vi "4p1_HW_Task1_pipoat.vi"() -> ()   [LabVIEW 2016]
uses:
  <vilib>/express/express arith-compare/Formula/XNode/ExpressFormulaBlockNode.xnode
panel:
  in  "Height":dbl
  out "Height of Fish":dbl
  in  "glass thickness (ft)":dbl
  in  "human distance from glass (ft)":dbl
  in  "fish distance from glass (ft)":dbl
  in  "reflective index of water":dbl
  in  "reflective index of glass":dbl
  in  "reflective index of air":dbl
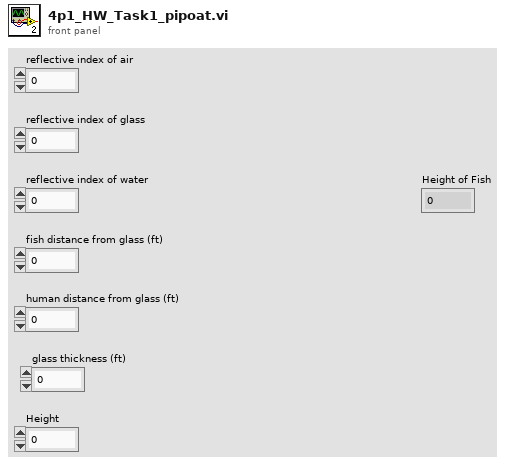
[diagram p1: front panel]
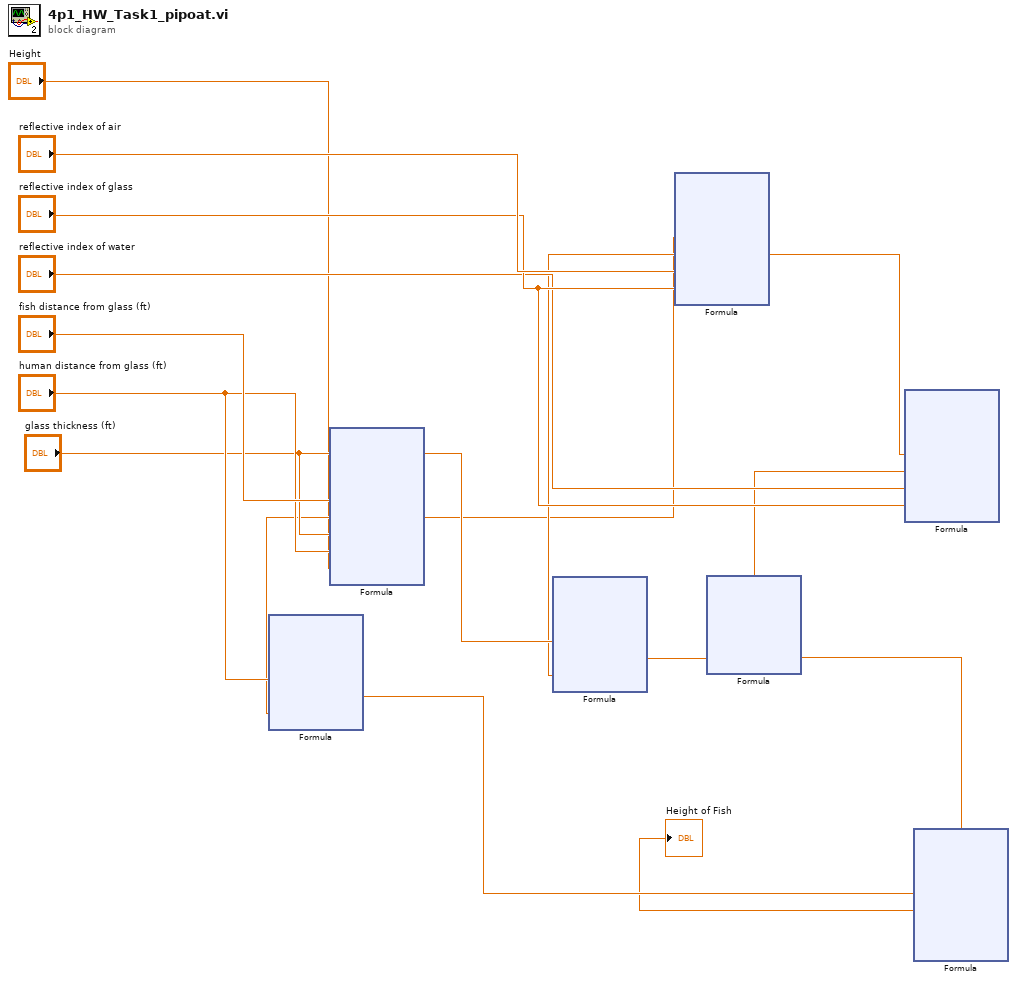
[diagram p0: block diagram]
diagram:
  n1 = xnode "Formula"("fish distance"="fish distance from glass (ft)", "glass thickness"="glass thickness (ft)", "human distance"="human distance from glass (ft)", "height"="Height") -> ("Result"=w2:dbl)  [unwired: 1 in, 1 out]
  n2 = xnode "Formula"("human distance"="human distance from glass (ft)", "tangent angle"=w2) -> ("Result"=w8:dbl)  [unwired: 1 in, 1 out]
  n3 = xnode "Formula"("tangent angle"=w2, "ref. index of air"="reflective index of air", "ref. index of glass"="reflective index of glass") -> ("Result"=w4:dbl)  [unwired: 1 in, 1 out]
  n4 = xnode "Formula"("glass thickness"="glass thickness (ft)", "angle B"=w4) -> ("Result"=w5:dbl)  [unwired: 1 in, 1 out]
  n5 = xnode "Formula"("Angle B"=w4, "ref. index of water"="reflective index of water", "ref. index of glass"="reflective index of glass") -> ("Result"=w3:dbl)  [unwired: 1 in, 1 out]
  n6 = xnode "Formula"("angle C"=w3) -> ("Result"=w7:dbl)  [unwired: 1 in, 1 out]
  n7 = xnode "Formula"("H1"=w8, "H2"=w5, "H3"=w7) -> ("Result"=→"Height of Fish":dbl)  [unwired: 1 in, 1 out]
